vi "Periodic Tasks.vi"(8 "error in":errorcluster) -> ()   [LabVIEW 2025]
doc: "This VI runs in parallel to other robot code. It can contain as many user-defined periodic loops as you need. These can carry out PID or other sorts of timed response."
uses:
  <vilib>/Analysis/coordinate.llb/Angle Units.ctl
  <vilib>/Analysis/coordinate.llb/Wrap Angle (scalar).vi
  <vilib>/Rock Robotics/WPI/ThirdParty/Phoenix-LabVIEW/Pigeon IMU/CTRE_PigeonIMU_GetYPR.vi
  <vilib>/Rock Robotics/Network Tables/NT Write Number.vi
  <vilib>/Rock Robotics/Network Tables/NT Write Numeric Array.vi
  <vilib>/Analysis/NI_AAL_Angle.lvlib
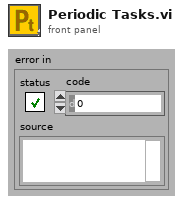
[diagram p1: front panel]
types:
  T1 = typedef "NI_AAL_Angle.lvlib/Angle Units.ctl" = i32
  T2 = typedef "CTRE_PigeonIMU_DeviceRef.ctl" = cluster{"DeviceStatus":errorcluster, "Device Number":u8, "Type":T3, "Device ID":u32, "Handle":u64, "UsageFrame":u32, "Library Path":path}
  T3 = typedef "CTRE_PigeonIMU_ConnectionType.ctl" = u32
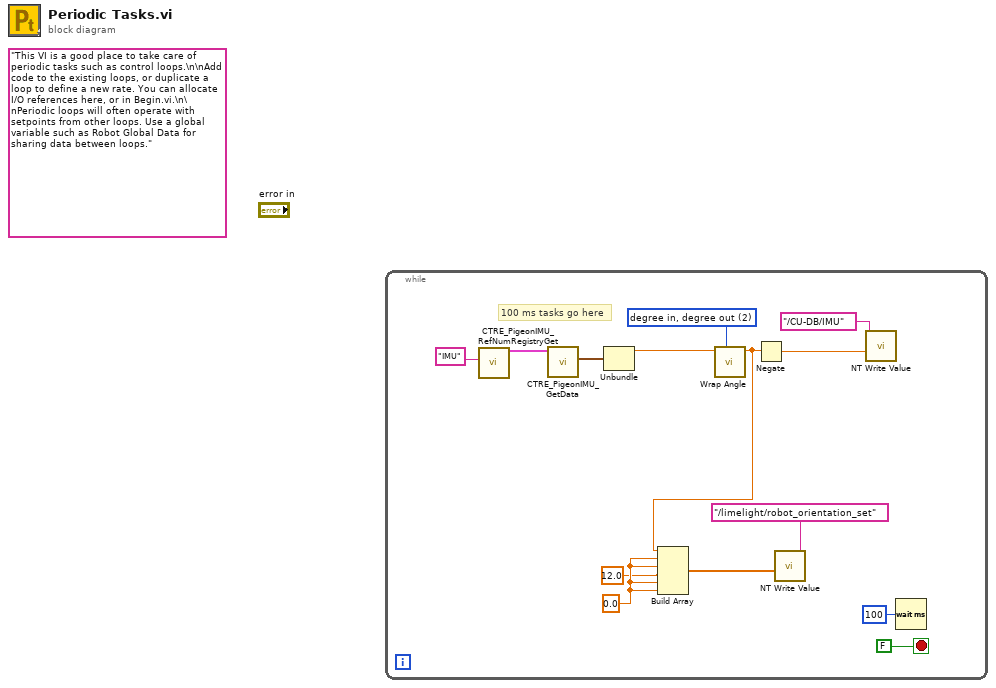
[diagram p0: block diagram]
diagram:
  (unwired) "This VI is a good place to take care of periodic tasks such as control loops.\n\nAdd code to the existing loops, or duplicate a loop to define a new rate. You can allocate I/O references here, or in Begin.vi.\n\nPeriodic loops will often operate with setpoints from other loops. Use a global variable such as Robot Global Data for sharing data between loops."
  n1 = while {
    stop <- FALSE stop-if-true
    w3 = 0.0 ("element")
    w11 = T1 2 items=["radian in, radian out", "radian in, degree out", "degree in, degree out", "degree in, radian out"] ("angle units")
    # "100 ms tasks go here"
    n2 = call <vilib>:"CTRE_PigeonIMU_RefNumRegistryGet.vi"("refnum name"="IMU") -> ("PigeonIMUDevRef"=w9:T2)  [unwired: 9 in, 1 out]
    n3 = call-poly <vilib>:"CTRE_PigeonIMU_GetData.vi"("PigeonIMUDevRef"=w9) -> ("Yaw Pitch Roll"=w8:cluster{"Yaw":dbl, "Pitch":dbl, "Roll":dbl})  [unwired: 8 in, 2 out]
    n4 = Unbundle(w8) -> ("Yaw"=w7:dbl)  [unwired: 2 out]
    n5 = call-poly <vilib>:"Wrap Angle.vi"("angle units"=w11, "angle in"=w7) -> ("angle out"=w1:dbl)  [unwired: 8 in, 1 out]
    n6 = Build Array(w1, w3, w3, 12.0 ("element"), w3, w3) -> (w5:dbl[])
    n7 = Negate(x=w1) -> (-x=w4:dbl)
    n8 = call-poly <vilib>:"NT Write Value.vi"("value"=w5, "name"="/limelight/robot_orientation_set") -> ()  [unwired: 9 in, 1 out]
    n9 = call-poly <vilib>:"NT Write Value.vi"("value"=w4, "name"="/CU-DB/IMU") -> ()  [unwired: 9 in, 1 out]
    n10 = Wait (ms)(milliseconds to wait=u32 100) -> ()  [unwired: 1 out]
  }
